vi "Dust_Type_Menu.vi"(8 "error in (no error)":errorcluster, 10 "Small?":bool, 11 "Enable":bool=TRUE) -> (0 "error out":errorcluster, 1 "Action Taken":T6(ring), 2 "Dust Properties":T3, 3 "Dust Info":T4 {"Batch" step=1; "Type" step=1; "Dust Source Builder:" items=["Keith Drake", "Nick Beaty", "Anthony Shu", "David James", "John Fontanese"]})   [LabVIEW 2015]
doc: "Displays a standard dialog box that prompts users to enter information, such as a user name and password.\n--------------------\n\nThis Express VI is configured as follows:\n\nMessage to Display to the User:Please Enter Experiment Settings Information For Database Storage.\nThe inputs are: \nNumber: Please Enter Group ID\nText Entry Box: Please Enter Tags:\nText Entry Box: Please Enter Experiment Description:"
uses:
  Controls/Dust_Properties.ctl
  Controls/source_builders.ctl
  Controls/dust_type_indicator.ctl
  Controls/Dust_list.ctl
  <vilib>/Utility/miscctls.llb/LVPointTypeDef.ctl
  <vilib>/Utility/error.llb/DialogType.ctl
  <userlib>/_OpenG.lib/array/array.llb/Remove Duplicates from 1D Array (String)__ogtk.vi
  <userlib>/_OpenG.lib/array/array.llb/Search 1D Array (String)__ogtk.vi
  <userlib>/_OpenG.lib/array/array.llb/Index 1D Array Elements (String)__ogtk.vi
  <vilib>/addons/database/_DB Variant To Data/Database Variant To Data.xnode
panel:
  out "Update Query":string
  out "Maxes Array":T1(array[cluster])
  out "All Dust Types":T2[](array[typedef])
  in  "Transfer":bool caption="OK2"
  in  "Controls":T4={"Dust info id"=0, "Integer Timestamp"=0, "Dust:"="", "Dust Source Builder:"=0, "Notes:"="", "Date of last dust source change:"=timestamp(0 s since 1904-01-01), "Initial Dust Mass:"=0.0, "Final Dust Mass:"=0.0, "Type"=0, "Batch"=1, "dust type id"=0, "Transferred?"=FALSE} {"Batch" min=1 max=2 step=1; "Type" min=1 max=1 step=1; "Dust Source Builder:" items=["Keith Drake", "Nick Beaty", "Anthony Shu", "David James", "John Fontanese"]}
  in  "Create New":bool caption="OK2"
  in  "Cancel":bool
  in  "Update":bool caption="OK1"
  # "Please Enter Dust Information For Storage in the CCLDAS Database."
  # "Dust Information"
  # "Dust Information"
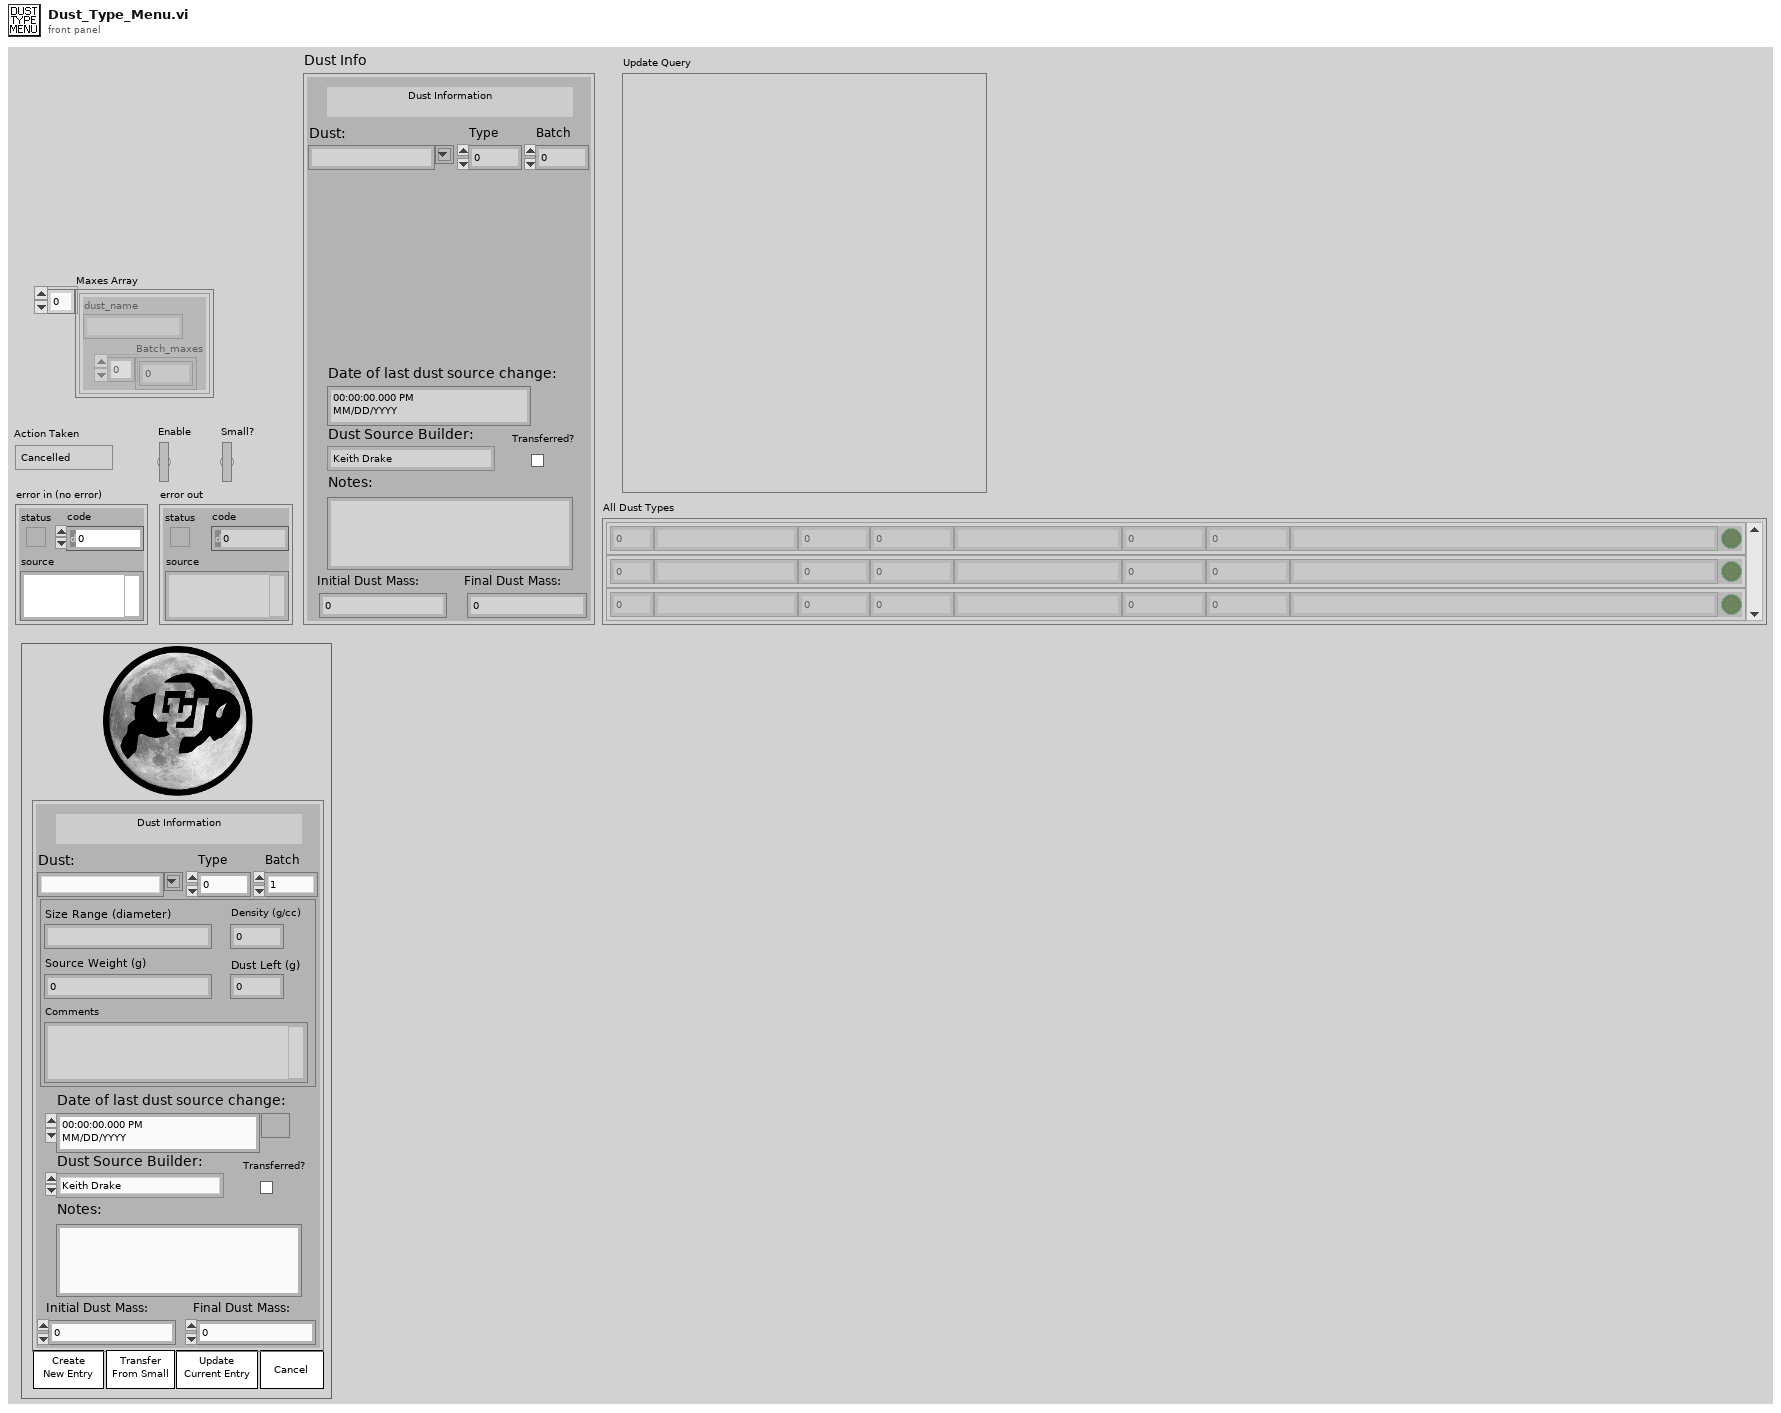
[diagram p1: front panel]
types:
  T1 = cluster{"dust_name":string, "Batch_maxes":i32[]}[]
  T2 = typedef "Dust_list.ctl" = cluster{"id_dust_type":i32, "dust_name":string, "dust_type":i32, "batch_no":i32, "dust_density":dbl, "source_weight":dbl, "size":string, "bottle_weight":dbl, "dust_mass":dbl, "comments":string, "Shoots?":bool}
  T3 = typedef "dust_type_indicator.ctl" = cluster{"id_dust_type":i32, "Size Range (diameter)":string, "Density (g/cc)":dbl, "Source Weight (g)":dbl, "Dust Left (g)":dbl, "Comments":string}
  T4 = typedef "Dust_Properties.ctl" = cluster{"Dust info id":u16, "Integer Timestamp":i64, "Dust:":string, "Dust Source Builder:":T5, "Notes:":string, "Date of last dust source change:":timestamp, "Initial Dust Mass:":dbl, "Final Dust Mass:":dbl, "Type":u16, "Batch":u16, "dust type id":u16, "Transferred?":bool}
  T5 = typedef "source_builders.ctl" = u16
  T6 = enum16{"Cancelled", "New", "Updated", "Transferred"}
  T7 = typedef "LVPointTypeDef.ctl" = cluster{"Horizontal":i16, "Vertical":i16}
  T8 = enum8{"Enabled", "Disabled", "Disabled and Grayed Out"}
  T9 = typedef "DialogType.ctl" = u16
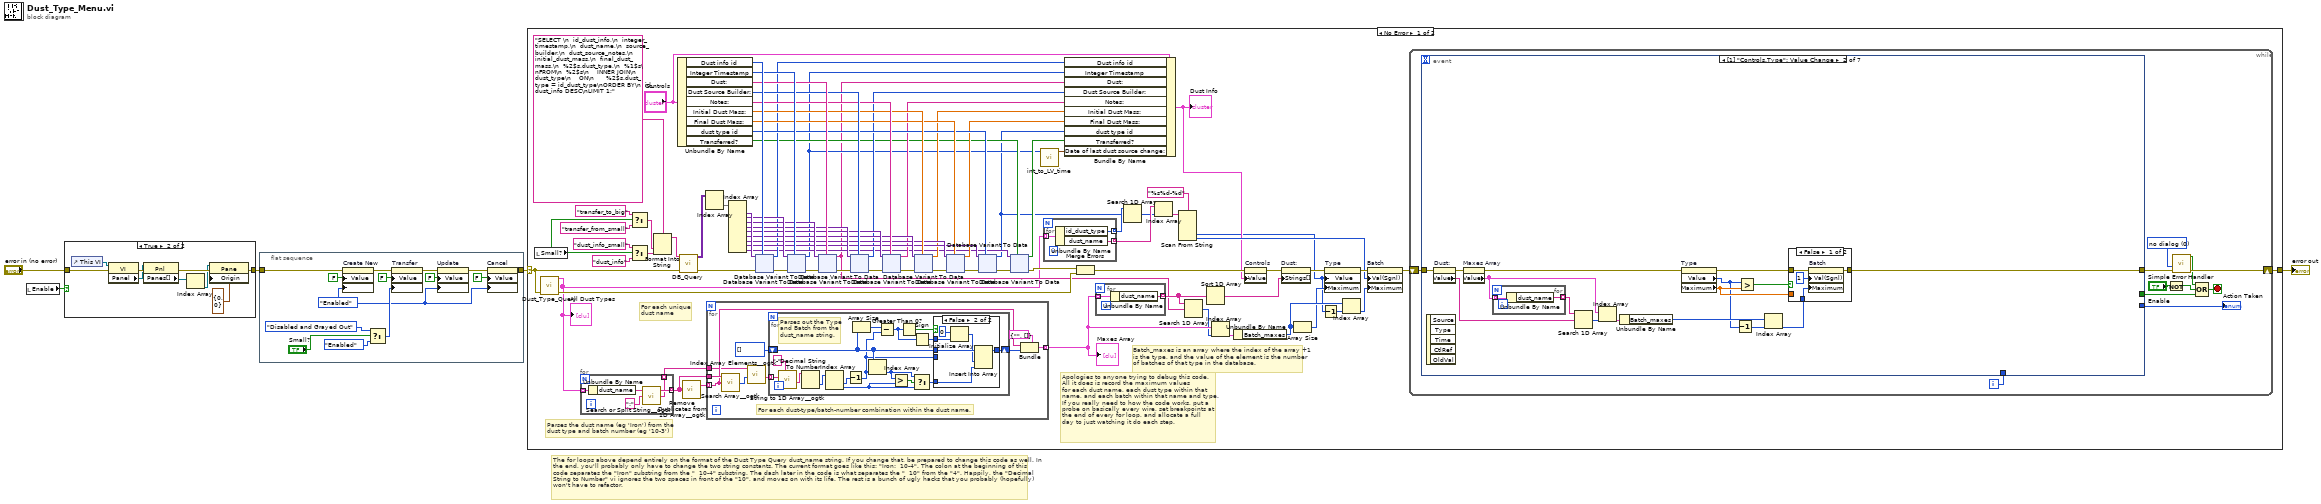
[diagram p0: block diagram]
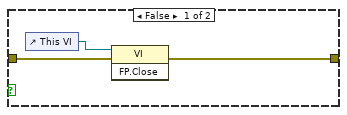
[diagram p2: hidden frame]
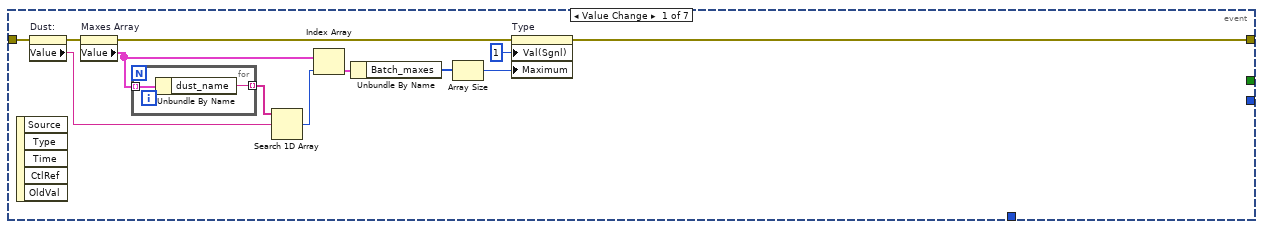
[diagram p3: hidden frame]
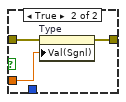
[diagram p4: hidden frame]
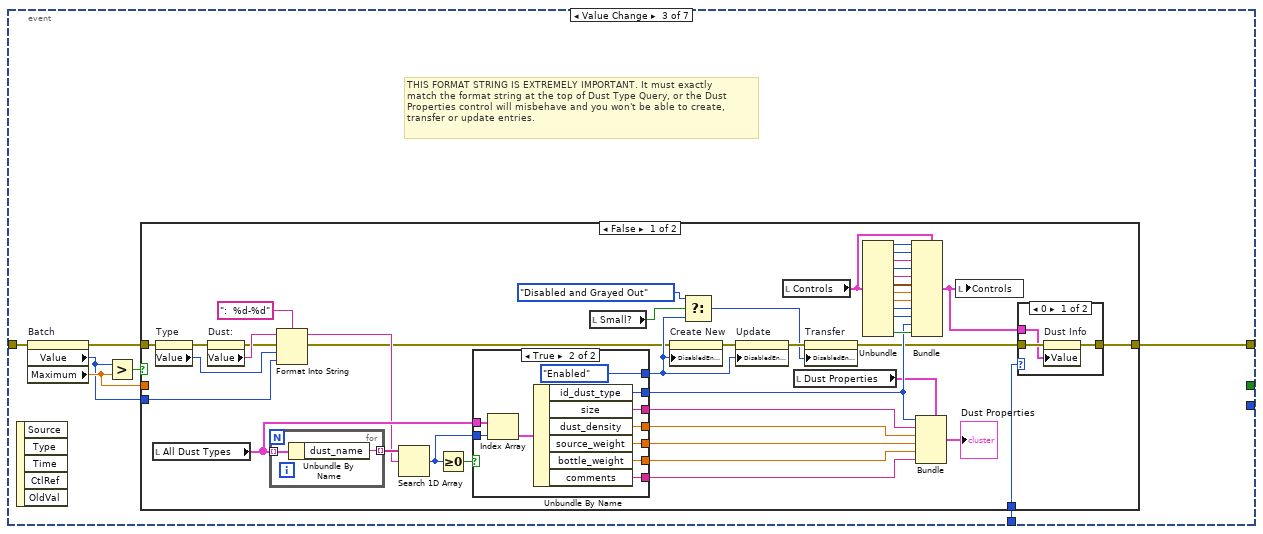
[diagram p5: hidden frame]
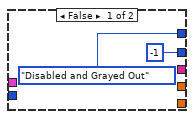
[diagram p7: hidden frame]
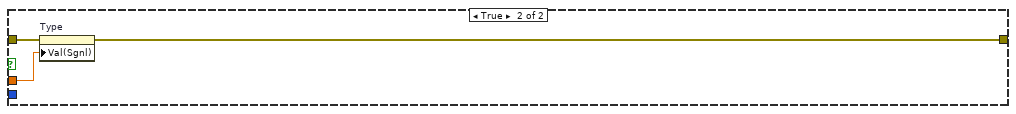
[diagram p8: hidden frame]
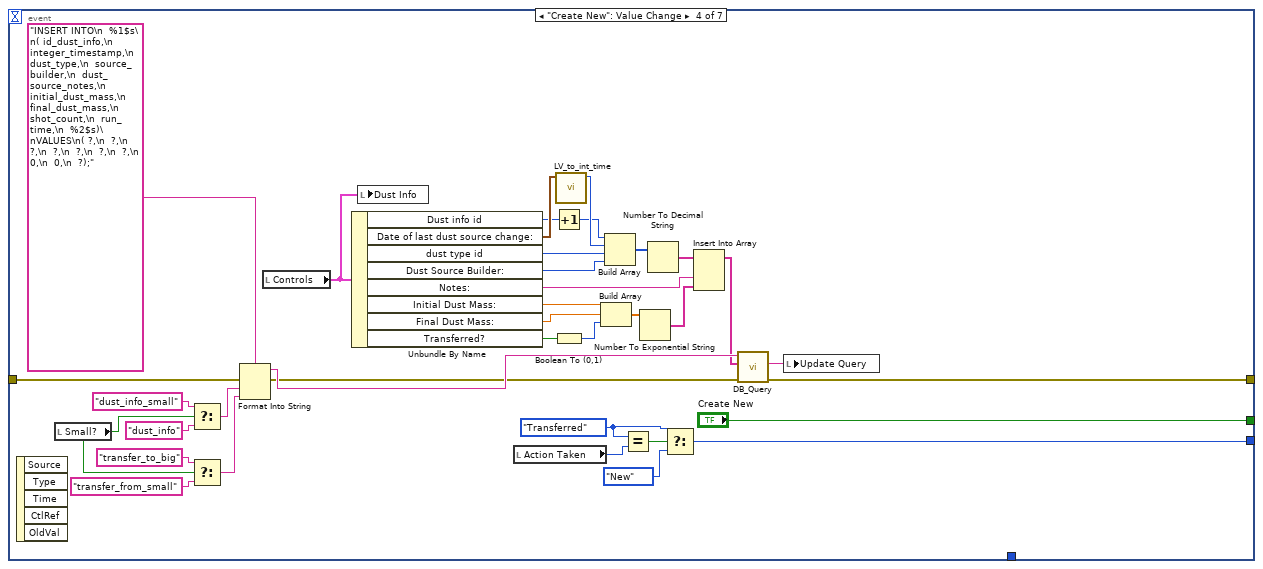
[diagram p9: hidden frame]
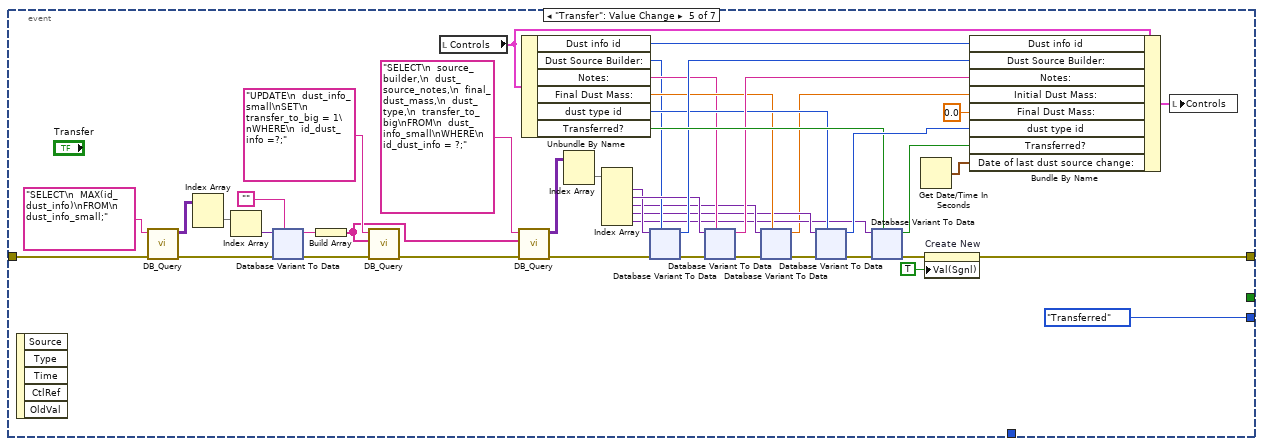
[diagram p10: hidden frame]
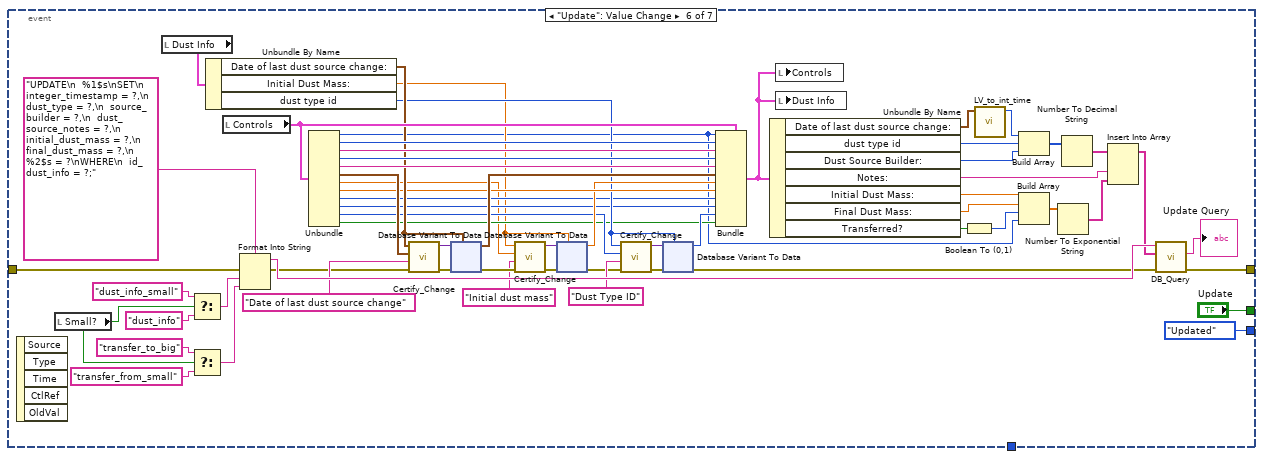
[diagram p11: hidden frame]
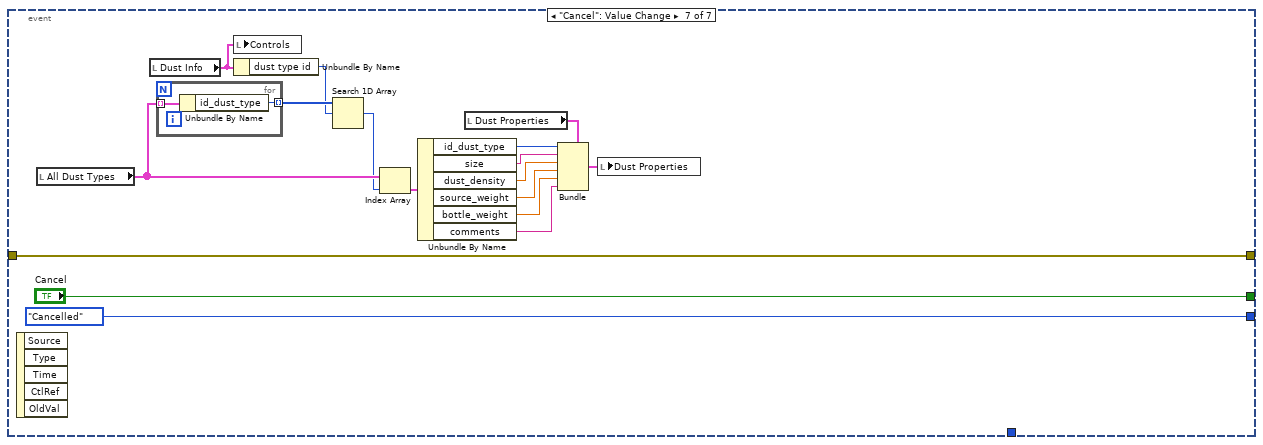
[diagram p12: hidden frame]
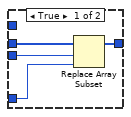
[diagram p13: hidden frame]
diagram:
  # "The for loops above depend entirely on the format of the Dust Type Query dust_name string. If you change that, be prepared to change this code as well. In\nthe end, you'll probably only have to change the two string constants. The current format goes like this: \"Iron:  10-4\". The colon at the beginning of this\ncode separates the \"Iron\" substring from the \"  10-4\" substring. The dash later in the code is what separates the \"  10\" from the \"4\". Happily, the \"Decimal\nString to Number\" vi ignores the two spaces in front of the \"10\", and moves on with its life. The rest is a bunch of ugly hacks that you probably (hopefully)\nwon't have to refactor."
  n1 = local read "Enable"() -> (w1:bool)
  n2 = case shown="True" w1 {
    tunnel: "error in (no error)" -> [w7 w10]
    tunnel: [w6 w9] -> w2
    frame False {
      n3 = control-ref of="This VI"() -> (w8:refnum<vi>)
      n4 = invoke class="VI" method="FP.Close"(reference=w8, error in=w7) -> (error out=w6:errorcluster)  [unwired: 1 in, 2 out]
    }
    frame True {
      n5 = control-ref of="This VI"() -> (w17:refnum<vi>)
      n6 = property class="VI"(reference=w17, error in=w10) -> (error out=w16:errorcluster, "Panel"=w15:refnum<vi>)  [unwired: 1 out]
      n7 = property class="Pnl"(reference=w15, error in=w16) -> (error out=w14:errorcluster, "Panes[]"=w13:refnum<vi>[])  [unwired: 1 out]
      n8 = Index Array(array=w13) -> (element=w12:refnum<vi>)  [unwired: 1 in]
      n9 = property class="Pane"(reference=w12, error in=w14, "Origin"=T7 {"Horizontal"=0, "Vertical"=0}) -> (error out=w9:errorcluster)  [unwired: 1 out]
    }
  }
  n10 = flat-sequence {
    tunnel: [w25] -> w3
    tunnel: w2 -> [w20]
    frame #0 {
      w18 = T8."Enabled" ("Disabled")
      n11 = property on="Create New" class="Bool (strict)"(error in=w20, "Value"=FALSE ("Create New"), "DisabledEnum"=w18) -> (error out=w26:errorcluster)  [unwired: 1 in, 1 out]
      n12 = Select(t=T8."Disabled and Grayed Out" ("Disabled"), s="Small?", f=T8."Enabled" ("Disabled")) -> (s? t:f=w19:T8)
      n13 = property on="Transfer" class="Bool (strict)"(error in=w26, "Value"=FALSE ("Transfer"), "DisabledEnum"=w19) -> (error out=w28:errorcluster)  [unwired: 1 in, 1 out]
      n14 = property on="Update" class="Bool (strict)"(error in=w28, "Value"=FALSE ("Update"), "DisabledEnum"=w18) -> (error out=w27:errorcluster)  [unwired: 1 in, 1 out]
      n15 = property on="Cancel" class="Bool (strict)"(error in=w27, "Value"=FALSE ("Cancel"), "DisabledEnum"=w18) -> (error out=w25:errorcluster)  [unwired: 1 in, 1 out]
    }
  }
  n16 = case shown="No Error" w3 {
    selector: w3 -> [w64 w1027]
    tunnel: [w55 w1027] -> w5
    frame No Error {
      # "Batch_maxes is an array where the index of the array +1\nis the type, and the value of the element is the number\nof batches of that type in the database."
      # "For each unique\ndust name"
      # "Parses the dust name (eg 'Iron') from the\ndust type and batch number (eg '10-3')"
      # "Apologies to anyone trying to debug this code.\nAll it does is record the maximum values\nfor each dust name, each dust type within that\nname, and each batch within that name and type.\nIf you really need to how the code works, put a\nprobe on basically every wire, set breakpoints at\nthe end of every for loop, and allocate a full\nday to just watching it do each step."
      n17 = local read "Small?"() -> (w102:bool)
      n18 = call "Dust_Type_Query.vi"("error in (no error)"=w64) -> ("error out"=w63:errorcluster, "Dust Type Array"=w43:T2[])  [unwired: 9 in]
      "All Dust Types" <- w43
      n19 = for {
        tunnel: w43 -> [w738] mode=indexing
        tunnel: [w736] -> w60 mode=indexing
        tunnel: [w734] -> w61 mode=indexing
        n20 = Unbundle By Name(w738) -> ("dust_name"=w735:string)
        n21 = call <userlib>:"Search or Split String__ogtk.vi"("search string/char (-)"=":", "string"=w735) -> ("substring after match"=w734:string, "substring before match"=w736:string)  [unwired: 1 in, 1 out]
      }
      n22 = Select(t="transfer_to_big", s=w102, f="transfer_from_small") -> (s? t:f=w103:string)
      n23 = Select(t="dust_info_small", s=w102, f="dust_info") -> (s? t:f=w107:string)
      n24 = Format Into String(format string="SELECT \n  id_dust_info,\n  integer_timestamp,\n  dust_name,\n  source_builder,\n  dust_source_notes,\n  initial_dust_mass,\n  final_dust_mass,\n  %2$s.dust_type,\n  %1$s\nFROM\n  %2$s\n    INNER JOIN\n  dust_type\n    ON\n      %2$s.dust_type = id_dust_type\nORDER BY\n  id_dust_info DESC\nLIMIT 1;" ("SQL query"), w103, w107) -> (resulting string=w106:string)  [unwired: 2 in, 1 out]
      n25 = Unbundle By Name("Controls") -> ("Dust info id"=w97:u16, "Integer Timestamp"=w94:i64, "Dust:"=w91:string, "Dust Source Builder:"=w89:T5, "Notes:"=w86:string, "Initial Dust Mass:"=w83:dbl, "Final Dust Mass:"=w79:dbl, "dust type id"=w76:u16, "Transferred?"=w68:bool)
      n26 = call "DB_Query.vi"("error in (no error)"=w64, "Parameterized Query"=w106) -> ("error out"=w101:errorcluster, "Results"=w100:variant[][])  [unwired: 7 in, 1 out]
      n27 = call-poly <userlib>:"Remove Duplicates from 1D Array__ogtk.vi"("Input Array"=w60) -> ("Output Array"=w62:string[])  [unwired: 1 out]
      n28 = Index Array(array=w100) -> (element=w99:variant[])  [unwired: 2 in]
      n29 = for {
        tunnel: w62 -> [w705] mode=indexing
        tunnel: w61 -> [w703]
        tunnel: w60 -> [w707]
        tunnel: [w699] -> w50 mode=indexing
        # "For each dust-type/batch-number combination within the dust name."
        n30 = call-poly <userlib>:"Search Array__ogtk.vi"("Array"=w707, "Element Data"=w705) -> ("Indices of Elements"=w704:i32[])  [unwired: 7 in]
        n31 = call-poly <userlib>:"Index Array Elements__ogtk.vi"("indices"=w704, "array"=w703) -> ("elements"=w702:string[])  [unwired: 9 in]
        n32 = for {
          tunnel: w702 -> [w720] mode=indexing
          shift-right: [w718] -> w700
          shift-left: i32[] [] ("array") -> [w713]
          # "Parses out the Type\nand Batch from the\ndust_name string."
          n33 = call <userlib>:"String to 1D Array__ogtk.vi"("delimiter (Tab)"="-", "string"=w720) -> ("Array of Strings"=w722:string[])  [unwired: 9 in]
          n34 = Decimal String To Number(string=w722) -> (number=w721:i32[])  [unwired: 2 in, 1 out]
          n35 = Index Array(array=w721) -> (element #1=w719:i32, element #2=w715:i32)  [unwired: 2 in]
          n36 = Decrement(x=w719) -> (x-1=w711:i32)
          n37 = Array Size(array=w713) -> (size(s)=w712:i32)
          n38 = Index Array(array=w713, index=w711) -> (element=w716:i32)
          n39 = Subtract(x=w712, y=w711) -> (x-y=w709:i32)
          n40 = Greater?(x=w716, y=w715) -> (0:w717:bool)
          n41 = Greater Than 0?(x=w709) -> (x > 0?=w710:bool)
          n42 = Select(t=w716, s=w717, f=w715) -> (s? t:f=w714:i32)
          n43 = Sign(1:w709) -> (0:w708:i32)
          n44 = case shown="False" w710 {
            tunnel: [w727 w733] -> w718
            tunnel: w713 -> [w726 w732]
            tunnel: w711 -> [w725 _]
            tunnel: w714 -> [w724 w731]
            tunnel: w708 -> [_ w730]
            frame True {
              n45 = Replace Array Subset(array=w726, new element=w724, index=w725) -> (w727:i32[])
            }
            frame False {
              n46 = Initialize Array(0 ("element"), w730) -> (w728:i32[])
              n47 = Insert Into Array(array=w732, new element #1=w728, new element #2=w731) -> (w733:i32[])  [unwired: 1 in]
            }
          }
        }
        n48 = Bundle(cluster=cluster{"dust_name":string, "Batch_maxes":i32[]} {"dust_name"="", "Batch_maxes"=[]}, "dust_name"=w705, "Batch_maxes"=w700) -> (w699:cluster{"dust_name":string, "Batch_maxes":i32[]})
      }
      "Maxes Array" <- w50
      n49 = Index Array(array=w99) -> (element #1=w98:variant, element #2=w95:variant, element #3=w92:variant, element #4=w88:variant, element #5=w85:variant, element #6=w82:variant, element #7=w80:variant, element #8=w77:variant, element #9=w66:variant)  [unwired: 9 in]
      n50 = xnode "Database Variant To Data"("database variant"=w98, "error in (no error)"=w101, "type"=w97) -> ("data"=w74:u16, "error out"=w96:errorcluster)
      n51 = xnode "Database Variant To Data"("database variant"=w95, "error in (no error)"=w96, "type"=w94) -> ("data"=w53:i64, "error out"=w93:errorcluster)
      n52 = xnode "Database Variant To Data"("database variant"=w92, "error in (no error)"=w93, "type"=w91) -> ("data"=w45:string, "error out"=w90:errorcluster)
      n53 = xnode "Database Variant To Data"("database variant"=w88, "error in (no error)"=w90, "type"=w89) -> ("data"=w73:T5, "error out"=w87:errorcluster)
      n54 = xnode "Database Variant To Data"("database variant"=w85, "error in (no error)"=w87, "type"=w86) -> ("data"=w72:string, "error out"=w84:errorcluster)
      n55 = xnode "Database Variant To Data"("database variant"=w82, "error in (no error)"=w84, "type"=w83) -> ("data"=w71:dbl, "error out"=w81:errorcluster)
      n56 = xnode "Database Variant To Data"("database variant"=w80, "error in (no error)"=w81, "type"=w79) -> ("data"=w70:dbl, "error out"=w78:errorcluster)
      n57 = xnode "Database Variant To Data"("database variant"=w77, "error in (no error)"=w78, "type"=w76) -> ("data"=w41:u16, "error out"=w69:errorcluster)
      n58 = xnode "Database Variant To Data"("database variant"=w66, "error in (no error)"=w69, "type"=w68) -> ("data"=w67:bool, "error out"=w65:errorcluster)
      n59 = call "int_to_LV_time.vi"("Integer Timestamp"=w53) -> ("time stamp"=w54:timestamp)  [unwired: 8 in, 1 out]
      n60 = for {
        tunnel: w43 -> [w113] mode=indexing
        tunnel: [w112] -> w42 mode=indexing
        tunnel: [w111] -> w40 mode=indexing
        n61 = Unbundle By Name(w113) -> ("id_dust_type"=w112:i32, "dust_name"=w111:string)
      }
      n62 = Bundle By Name(cluster="Controls", "Dust info id"=w74, "Integer Timestamp"=w53, "Dust:"=w45, "Dust Source Builder:"=w73, "Notes:"=w72, "Initial Dust Mass:"=w71, "Final Dust Mass:"=w70, "dust type id"=w41, "Transferred?"=w67, "Date of last dust source change:"=w54) -> (w33:T4)
      "Dust Info" <- w33
      n63 = Merge Errors(w65, w63) -> (w34:errorcluster)
      n64 = for {
        tunnel: w50 -> [w698] mode=indexing
        tunnel: [w697] -> w49 mode=indexing
        n65 = Unbundle By Name(w698) -> ("dust_name"=w697:string)
      }
      n66 = Search 1D Array(1D array=w42, element=w41) -> (index of element=w39:i32)  [unwired: 1 in]
      n67 = Index Array(array=w40, index=w39) -> (element=w38:string)
      n68 = Scan From String(format string="%s%d-%d", input string=w38) -> (output 2=w32:i32, output 3=w36:i32)  [unwired: 6 in, 3 out]
      n69 = Search 1D Array(1D array=w49, element=w45) -> (index of element=w48:i32)  [unwired: 1 in]
      n70 = Sort 1D Array(array=w49) -> (sorted array=w52:string[])
      n71 = Index Array(array=w50, index=w48) -> (element=w59:cluster{"dust_name":string, "Batch_maxes":i32[]})
      n72 = Unbundle By Name(w59) -> ("Batch_maxes"=w58:i32[])
      n73 = property on="Controls" class="Clust (strict)"(error in=w34, "Value"=w33) -> (error out=w35:errorcluster)  [unwired: 1 in, 1 out]
      n74 = property on="Dust:" class="CmbBox"(error in=w35, "Strings[]"=w52) -> (error out=w56:errorcluster)  [unwired: 1 in, 1 out]
      n75 = Array Size(array=w58) -> (size(s)=w46:i32)
      n76 = Decrement(x=w32) -> (x-1=w47:i32)
      n77 = property on="Type" class="DigNum (strict)"(error in=w56, "Value"=w32, "Maximum"=w46) -> (error out=w57:errorcluster)  [unwired: 1 in, 1 out]
      n78 = Index Array(array=w58, index=w47) -> (element=w51:i32)
      n79 = property on="Batch" class="DigNum (strict)"(error in=w57, "Val(Sgnl)"=w36, "Maximum"=w51) -> (error out=w44:errorcluster)  [unwired: 1 in, 1 out]
      n80 = while {
        shift-right: [w120] -> w55
        shift-left: w44 -> [w124]
        i -> [w114]
        stop <- w118 stop-if-true
        w119 = T9 0 items=["no dialog", "OK message", "continue or stop message", "OK message + warnings", "continue/stop + warnings"] ("type of dialog (OK msg:1)")
        n81 = event shown="[1] \"Controls.Type\": Value Change" {
          selector: _ -> [_ _ _ _ _ _ _]
          dyn-events: _ -> [_ _ _ _ _ _ _]
          timeout: _ -> [_ _ _ _ _ _ _]
          tunnel: w124 -> [w136 w148 w167 w245 w281 w558 w693]
          tunnel: [w125 w145 w166 w247 w282 w544 w693] -> w123
          tunnel: [_ _ _ "Create New" _ "Update" "Cancel"] -> w122
          tunnel: [_ _ _ w235 T6."Transferred" ("Action Taken") T6."Updated" ("Action Taken") T6."Cancelled" ("Action Taken")] -> w121
          tunnel: w114 -> [_ _ w164 _ _ _ _]
          event Value Change {
            n82 = event-data() -> ()  [unwired: 1 in, 5 out]
            n83 = property on="Dust:" class="CmbBox"(error in=w136) -> (error out=w135:errorcluster, "Value"=w126:string)  [unwired: 1 in, 1 out]
            n84 = property on="Maxes Array" class="Arr (strict)"(error in=w135) -> (error out=w134:errorcluster, "Value"=w131:T1)  [unwired: 1 in, 1 out]
            n85 = for {
              tunnel: w131 -> [w138] mode=indexing
              tunnel: [w137] -> w133 mode=indexing
              n86 = Unbundle By Name(w138) -> ("dust_name"=w137:string)
            }
            n87 = Search 1D Array(1D array=w133, element=w126) -> (index of element=w127:i32)  [unwired: 1 in]
            n88 = Index Array(array=w131, index=w127) -> (element=w130:cluster{"dust_name":string, "Batch_maxes":i32[]})
            n89 = Unbundle By Name(w130) -> ("Batch_maxes"=w129:i32[])
            n90 = Array Size(array=w129) -> (size(s)=w128:i32)
            n91 = property on="Type" class="DigNum (strict)"(error in=w134, "Val(Sgnl)"=u16 1 ("Value"), "Maximum"=w128) -> (error out=w125:errorcluster)  [unwired: 1 in, 1 out]
          }
          event Value Change {
            n92 = event-data() -> ()  [unwired: 1 in, 5 out]
            n93 = property on="Dust:" class="CmbBox"(error in=w148) -> (error out=w154:errorcluster, "Value"=w152:string)  [unwired: 1 in, 1 out]
            n94 = property on="Maxes Array" class="Arr (strict)"(error in=w154) -> (error out=w142:errorcluster, "Value"=w150:T1)  [unwired: 1 in, 1 out]
            n95 = for {
              tunnel: w150 -> [w163] mode=indexing
              tunnel: [w162] -> w153 mode=indexing
              n96 = Unbundle By Name(w163) -> ("dust_name"=w162:string)
            }
            n97 = Search 1D Array(1D array=w153, element=w152) -> (index of element=w151:i32)  [unwired: 1 in]
            n98 = Index Array(array=w150, index=w151) -> (element=w149:cluster{"dust_name":string, "Batch_maxes":i32[]})
            n99 = Unbundle By Name(w149) -> ("Batch_maxes"=w141:i32[])
            n100 = property on="Type" class="DigNum (strict)"(error in=w142) -> (error out=w147:errorcluster, "Value"=w140:u16, "Maximum"=w146:dbl)  [unwired: 1 in, 1 out]
            n101 = Decrement(x=w140) -> (x-1=w139:u16)
            n102 = Greater?(x=w140, y=w146) -> (0:w144:bool)
            n103 = Index Array(array=w141, index=w139) -> (element=w143:i32)
            n104 = case shown="False" w144 {
              tunnel: w147 -> [w157 w161]
              tunnel: w146 -> [_ w160]
              tunnel: [w156 w159] -> w145
              tunnel: w143 -> [w155 _]
              frame False {
                n105 = property on="Batch" class="DigNum (strict)"(error in=w157, "Val(Sgnl)"=u16 1 ("Value (Signaling)"), "Maximum"=w155) -> (error out=w156:errorcluster)  [unwired: 1 in, 1 out]
              }
              frame True {
                n106 = property on="Type" class="DigNum (strict)"(error in=w161, "Val(Sgnl)"=w160) -> (error out=w159:errorcluster)  [unwired: 1 in, 1 out]
              }
            }
          }
          event Value Change {
            # "THIS FORMAT STRING IS EXTREMELY IMPORTANT. It must exactly\nmatch the format string at the top of Dust Type Query, or the Dust\nProperties control will misbehave and you won't be able to create,\ntransfer or update entries."
            n107 = event-data() -> ()  [unwired: 1 in, 5 out]
            n108 = property on="Batch" class="DigNum (strict)"(error in=w167) -> (error out=w170:errorcluster, "Value"=w165:u16, "Maximum"=w169:dbl)  [unwired: 1 in, 1 out]
            n109 = Greater?(x=w165, y=w169) -> (0:w168:bool)
            n110 = case shown="False" w168 {
              tunnel: w170 -> [w208 w234]
              tunnel: w169 -> [_ w233]
              tunnel: [w174 w232] -> w166
              tunnel: w165 -> [w207 _]
              tunnel: w164 -> [w171 _]
              frame False {
                n111 = local read "All Dust Types"() -> (w213:T2[])
                n112 = property on="Type" class="DigNum (strict)"(error in=w208) -> (error out=w209:errorcluster, "Value"=w205:u16)  [unwired: 1 in, 1 out]
                n113 = property on="Dust:" class="CmbBox"(error in=w209) -> (error out=w177:errorcluster, "Value"=w206:string)  [unwired: 1 in, 1 out]
                n114 = for {
                  tunnel: w213 -> [w231] mode=indexing
                  tunnel: [w230] -> w212 mode=indexing
                  n115 = Unbundle By Name(w231) -> ("dust_name"=w230:string)
                }
                n116 = Format Into String(format string=":  %d-%d", initial string=w206, error in=w177, w205, w207) -> (resulting string=w210:string, error out=w176:errorcluster)
                n117 = Search 1D Array(1D array=w212, element=w210) -> (index of element=w185:i32)  [unwired: 1 in]
                n118 = Greater Or Equal To 0?(x=w185) -> (x >= 0?=w186:bool)
                n119 = case shown="True" w186 {
                  tunnel: w213 -> [_ w228]
                  tunnel: w185 -> [_ w227]
                  tunnel: [_ w226] -> w204
                  tunnel: [_ w225] -> w203
                  tunnel: [_ w224] -> w202
                  tunnel: [_ w223] -> w201
                  tunnel: [_ w222] -> w200
                  tunnel: [-1 ("id_dust_type") w221] -> w187
                  tunnel: [T8."Disabled and Grayed Out" ("Disabled") T8."Enabled" ("Disabled")] -> w179
                  frame False {
                  }
                  frame True {
                    n120 = Index Array(array=w228, index=w227) -> (element=w229:T2)
                    n121 = Unbundle By Name(w229) -> ("id_dust_type"=w221:i32, "size"=w226:string, "dust_density"=w225:dbl, "source_weight"=w224:dbl, "bottle_weight"=w223:dbl, "comments"=w222:string)
                  }
                }
                n122 = local read "Small?"() -> (w180:bool)
                n123 = property on="Create New" class="Bool (strict)"(error in=w176, "DisabledEnum"=w179) -> (error out=w182:errorcluster)  [unwired: 1 in, 1 out]
                n124 = Select(t=T8."Disabled and Grayed Out" ("Disabled"), s=w180, f=w179) -> (s? t:f=w178:T8)
                n125 = property on="Update" class="Bool (strict)"(error in=w182, "DisabledEnum"=w179) -> (error out=w183:errorcluster)  [unwired: 1 in, 1 out]
                n126 = local read "Controls"() -> (w199:T4)
                n127 = local read "Dust Properties"() -> (w184:T3)
                n128 = property on="Transfer" class="Bool (strict)"(error in=w183, "DisabledEnum"=w178) -> (error out=w172:errorcluster)  [unwired: 1 in, 1 out]
                n129 = Unbundle(w199) -> ("Dust info id"=w198:u16, "Integer Timestamp"=w197:i64, "Dust:"=w196:string, "Dust Source Builder:"=w195:T5, "Notes:"=w194:string, "Date of last dust source change:"=w193:timestamp, "Initial Dust Mass:"=w192:dbl, "Final Dust Mass:"=w191:dbl, "Type"=w190:u16, "Batch"=w189:u16, "Transferred?"=w188:bool)  [unwired: 1 out]
                n130 = Bundle(cluster=w199, "Dust info id"=w198, "Integer Timestamp"=w197, "Dust:"=w196, "Dust Source Builder:"=w195, "Notes:"=w194, "Date of last dust source change:"=w193, "Initial Dust Mass:"=w192, "Final Dust Mass:"=w191, "Type"=w190, "Batch"=w189, "dust type id"=w187, "Transferred?"=w188) -> (w173:T4)
                n131 = Bundle(cluster=w184, "id_dust_type"=w187, "Size Range (diameter)"=w204, "Density (g/cc)"=w203, "Source Weight (g)"=w202, "Dust Left (g)"=w201, "Comments"=w200) -> (→"Dust Properties":T3)
                n132 = local write "Controls"(w173) -> ()
                n133 = case shown="0" w171 {
                  tunnel: w172 -> [w216 w217]
                  tunnel: [w215 w217] -> w174
                  tunnel: w173 -> [w214 _]
                  frame 0 {
                    n134 = property on="Dust Info" class="Clust (strict)"(error in=w216, "Value"=w214) -> (error out=w215:errorcluster)  [unwired: 1 in, 1 out]
                  }
                  frame Default {
                  }
                }
              }
              frame True {
                n135 = property on="Type" class="DigNum (strict)"(error in=w234, "Val(Sgnl)"=w233) -> (error out=w232:errorcluster)  [unwired: 1 in, 1 out]
              }
            }
          }
          event "Create New": Value Change {
            w237 = T6."Transferred" ("Action Taken")
            n136 = event-data() -> ()  [unwired: 1 in, 5 out]
            n137 = local read "Small?"() -> (w267:bool)
            n138 = Select(t="dust_info_small", s=w267, f="dust_info") -> (s? t:f=w264:string)
            n139 = Select(t="transfer_to_big", s=w267, f="transfer_from_small") -> (s? t:f=w263:string)
            n140 = Format Into String(format string="INSERT INTO\n  %1$s\n( id_dust_info,\n  integer_timestamp,\n  dust_type,\n  source_builder,\n  dust_source_notes,\n  initial_dust_mass,\n  final_dust_mass,\n  shot_count,\n  run_time,\n  %2$s)\nVALUES\n( ?,\n  ?,\n  ?,\n  ?,\n  ?,\n  ?,\n  ?,\n  0,\n  0,\n  ?);", error in=w245, w264, w263) -> (resulting string=w268:string, error out=w243:errorcluster)  [unwired: 1 in]
            n141 = local read "Controls"() -> (w244:T4)
            n142 = Unbundle By Name(w244) -> ("Dust info id"=w242:u16, "Date of last dust source change:"=w262:timestamp, "dust type id"=w259:u16, "Dust Source Builder:"=w248:T5, "Notes:"=w249:string, "Initial Dust Mass:"=w257:dbl, "Final Dust Mass:"=w256:dbl, "Transferred?"=w261:bool)
            n143 = local write "Dust Info"(w244) -> ()
            n144 = local read "Action Taken"() -> (w238:T6)
            n145 = Increment(x=w242) -> (x+1=w241:u16)
            n146 = Boolean To (0,1)(Boolean=w261) -> (0, 1=w255:i16)
            n147 = call "LV_to_int_time.vi"("Time Stamp"=w262) -> ("Integer Time"=w260:i64)  [unwired: 8 in, 1 out]
            n148 = Build Array(w257, w256, w255) -> (w254:dbl[])
            n149 = Build Array(w241, w260, w259, w248) -> (w258:i64[])
            n150 = Equal?(x=w237, y=w238) -> (x = y?=w239:bool)
            n151 = Number To Exponential String(number=w254) -> (E-format string=w252:string[])  [unwired: 3 in]
            n152 = Number To Decimal String(number=w258) -> (decimal integer string=w253:string[])  [unwired: 1 in]
            n153 = Select(t=w237, s=w239, f=T6."New" ("Action Taken")) -> (s? t:f=w235:T6)
            n154 = Insert Into Array(array=w253, new element #1=w249, new element #2=w252) -> (w251:string[])  [unwired: 1 in]
            n155 = call "DB_Query.vi"("error in (no error)"=w243, "Parameters"=w251, "Parameterized Query"=w268) -> ("error out"=w247:errorcluster, "Query in Standard Format"=w246:string)  [unwired: 6 in, 1 out]
            n156 = local write "Update Query"(w246) -> ()
          }
          event "Transfer": Value Change {
            n157 = event-data() -> ()  [unwired: 1 in, 5 out]
            n158 = call "DB_Query.vi"("error in (no error)"=w281, "Parameterized Query"="SELECT\n  MAX(id_dust_info)\nFROM\n  dust_info_small;") -> ("error out"=w275:errorcluster, "Results"=w279:variant[][])  [unwired: 7 in, 1 out]
            n159 = Index Array(array=w279) -> (element=w278:variant[])  [unwired: 2 in]
            n160 = Index Array(array=w278) -> (element=w277:variant)  [unwired: 1 in]
            n161 = xnode "Database Variant To Data"("database variant"=w277, "error in (no error)"=w275, "type"="") -> ("data"=w273:string, "error out"=w274:errorcluster)
            n162 = Build Array(w273) -> (w272:string[])
            n163 = call "DB_Query.vi"("error in (no error)"=w274, "Parameters"=w272, "Parameterized Query"="UPDATE\n  dust_info_small\nSET\n  transfer_to_big = 1\nWHERE\n  id_dust_info =?;") -> ("error out"=w310:errorcluster)  [unwired: 6 in, 2 out]
            n164 = local read "Controls"() -> (w294:T4)
            n165 = call "DB_Query.vi"("error in (no error)"=w310, "Parameters"=w272, "Parameterized Query"="SELECT\n  source_builder,\n  dust_source_notes,\n  final_dust_mass,\n  dust_type,\n  transfer_to_big\nFROM\n  dust_info_small\nWHERE\n  id_dust_info = ?;") -> ("error out"=w285:errorcluster, "Results"=w312:variant[][])  [unwired: 6 in, 1 out]
            n166 = Unbundle By Name(w294) -> ("Dust info id"=w271:u16, "Dust Source Builder:"=w296:T5, "Notes:"=w299:string, "Final Dust Mass:"=w301:dbl, "dust type id"=w303:u16, "Transferred?"=w307:bool)
            n167 = Index Array(array=w312) -> (element=w295:variant[])  [unwired: 2 in]
            n168 = Index Array(array=w295) -> (element #1=w297:variant, element #2=w300:variant, element #3=w290:variant, element #4=w289:variant, element #5=w288:variant)  [unwired: 5 in]
            n169 = xnode "Database Variant To Data"("database variant"=w297, "error in (no error)"=w285, "type"=w296) -> ("data"=w304:T5, "error out"=w298:errorcluster)
            n170 = xnode "Database Variant To Data"("database variant"=w300, "error in (no error)"=w298, "type"=w299) -> ("data"=w305:string, "error out"=w291:errorcluster)
            n171 = xnode "Database Variant To Data"("database variant"=w290, "error in (no error)"=w291, "type"=w301) -> ("data"=w287:dbl, "error out"=w302:errorcluster)
            n172 = xnode "Database Variant To Data"("database variant"=w289, "error in (no error)"=w302, "type"=w303) -> ("data"=w309:u16, "error out"=w306:errorcluster)
            n173 = xnode "Database Variant To Data"("database variant"=w288, "error in (no error)"=w306, "type"=w307) -> ("data"=w308:bool, "error out"=w284:errorcluster)
            n174 = Get Date/Time In Seconds() -> (seconds since 1Jan1904=w293:timestamp)
            n175 = property on="Create New" class="Bool (strict)"(error in=w284, "Val(Sgnl)"=TRUE ("Value (Signaling)")) -> (error out=w282:errorcluster)  [unwired: 1 in, 1 out]
            n176 = Bundle By Name(cluster=w294, "Dust info id"=w271, "Dust Source Builder:"=w304, "Notes:"=w305, "Initial Dust Mass:"=w287, "Final Dust Mass:"=0.0, "dust type id"=w309, "Transferred?"=w308, "Date of last dust source change:"=w293) -> (w292:T4)
            n177 = local write "Controls"(w292) -> ()
          }
          event "Update": Value Change {
            n178 = event-data() -> ()  [unwired: 1 in, 5 out]
            n179 = local read "Small?"() -> (w564:bool)
            n180 = local read "Dust Info"() -> (w540:T4)
            n181 = Select(t="dust_info_small", s=w564, f="dust_info") -> (s? t:f=w560:string)
            n182 = Select(t="transfer_to_big", s=w564, f="transfer_from_small") -> (s? t:f=w559:string)
            n183 = Unbundle By Name(w540) -> ("Date of last dust source change:"=w529:timestamp, "Initial Dust Mass:"=w510:dbl, "dust type id"=w518:u16)
            n184 = local read "Controls"() -> (w535:T4)
            n185 = Format Into String(format string="UPDATE\n  %1$s\nSET\n  integer_timestamp = ?,\n  dust_type = ?,\n  source_builder = ?,\n  dust_source_notes = ?,\n  initial_dust_mass = ?,\n  final_dust_mass = ?,\n  %2$s = ?\nWHERE\n  id_dust_info = ?;", error in=w558, w560, w559) -> (resulting string=w566:string, error out=w533:errorcluster)  [unwired: 1 in]
            n186 = Unbundle(w535) -> ("Dust info id"=w508:u16, "Integer Timestamp"=w539:i64, "Dust:"=w538:string, "Dust Source Builder:"=w537:T5, "Notes:"=w536:string, "Date of last dust source change:"=w532:timestamp, "Initial Dust Mass:"=w509:dbl, "Final Dust Mass:"=w524:dbl, "Type"=w516:u16, "Batch"=w515:u16, "dust type id"=w517:u16, "Transferred?"=w513:bool)
            n187 = call "Certify_Change.vi"("error in (no error)"=w533, "Variable Name"="Date of last dust source change", "New Value"=w532, "Default Value"=w529) -> ("error out"=w531:errorcluster, "Value Out"=w530:variant)  [unwired: 6 in]
            n188 = xnode "Database Variant To Data"("database variant"=w530, "error in (no error)"=w531, "type"=w529) -> ("data"=w528:timestamp, "error out"=w525:errorcluster)
            n189 = call "Certify_Change.vi"("error in (no error)"=w525, "Variable Name"="Initial dust mass", "New Value"=w509, "Default Value"=w510) -> ("error out"=w526:errorcluster, "Value Out"=w527:variant)  [unwired: 6 in]
            n190 = xnode "Database Variant To Data"("database variant"=w527, "error in (no error)"=w526, "type"=w510) -> ("data"=w522:dbl, "error out"=w512:errorcluster)
            n191 = call "Certify_Change.vi"("error in (no error)"=w512, "Variable Name"="Dust Type ID", "New Value"=w517, "Default Value"=w518) -> ("error out"=w520:errorcluster, "Value Out"=w519:variant)  [unwired: 6 in]
            n192 = xnode "Database Variant To Data"("database variant"=w519, "error in (no error)"=w520, "type"=w518) -> ("data"=w514:u16, "error out"=w511:errorcluster)
            n193 = Bundle(cluster=w535, "Dust info id"=w508, "Integer Timestamp"=w539, "Dust:"=w538, "Dust Source Builder:"=w537, "Notes:"=w536, "Date of last dust source change:"=w528, "Initial Dust Mass:"=w522, "Final Dust Mass:"=w524, "Type"=w516, "Batch"=w515, "dust type id"=w514, "Transferred?"=w513) -> (w507:T4)
            n194 = Unbundle By Name(w507) -> ("Date of last dust source change:"=w557:timestamp, "dust type id"=w554:u16, "Dust Source Builder:"=w541:T5, "Notes:"=w542:string, "Initial Dust Mass:"=w552:dbl, "Final Dust Mass:"=w551:dbl, "Transferred?"=w556:bool)
            n195 = local write "Controls"(w507) -> ()
            n196 = local write "Dust Info"(w507) -> ()
            n197 = Boolean To (0,1)(Boolean=w556) -> (0, 1=w550:i16)
            n198 = call "LV_to_int_time.vi"("Time Stamp"=w557) -> ("Integer Time"=w555:i64)  [unwired: 8 in, 1 out]
            n199 = Build Array(w555, w554, w541) -> (w553:i64[])
            n200 = Build Array(w552, w551, w550, w508) -> (w549:dbl[])
            n201 = Number To Exponential String(number=w549) -> (E-format string=w547:string[])  [unwired: 3 in]
            n202 = Number To Decimal String(number=w553) -> (decimal integer string=w548:string[])  [unwired: 1 in]
            n203 = Insert Into Array(array=w548, new element #1=w542, new element #2=w547) -> (w546:string[])  [unwired: 1 in]
            n204 = call "DB_Query.vi"("error in (no error)"=w511, "Parameters"=w546, "Parameterized Query"=w566) -> ("error out"=w544:errorcluster, "Query in Standard Format"=→"Update Query":string)  [unwired: 6 in, 1 out]
          }
          event "Cancel": Value Change {
            n205 = event-data() -> ()  [unwired: 1 in, 5 out]
            n206 = local read "All Dust Types"() -> (w682:T2[])
            n207 = local read "Dust Info"() -> (w678:T4)
            n208 = for {
              tunnel: w682 -> [w696] mode=indexing
              tunnel: [w695] -> w681 mode=indexing
              n209 = Unbundle By Name(w696) -> ("id_dust_type"=w695:i32)
            }
            n210 = local write "Controls"(w678) -> ()
            n211 = Unbundle By Name(w678) -> ("dust type id"=w680:u16)
            n212 = Search 1D Array(1D array=w681, element=w680) -> (index of element=w679:i32)  [unwired: 1 in]
            n213 = Index Array(array=w682, index=w679) -> (element=w692:T2)
            n214 = Unbundle By Name(w692) -> ("id_dust_type"=w683:i32, "size"=w684:string, "dust_density"=w685:dbl, "source_weight"=w686:dbl, "bottle_weight"=w687:dbl, "comments"=w688:string)
            n215 = local read "Dust Properties"() -> (w691:T3)
            n216 = Bundle(cluster=w691, "id_dust_type"=w683, "Size Range (diameter)"=w684, "Density (g/cc)"=w685, "Source Weight (g)"=w686, "Dust Left (g)"=w687, "Comments"=w688) -> (w690:T3)
            n217 = local write "Dust Properties"(w690) -> ()
          }
        }
        "Action Taken" <- w121
        n218 = Not(x="Enable") -> (.not. x?=w115:bool)
        n219 = call <vilib>:"Simple Error Handler.vi"("type of dialog (OK msg:1)"=w119, "error in (no error)"=w123) -> ("error?"=w117:bool, "error out"=w120:errorcluster)  [unwired: 3 in, 3 out]
        n220 = Compound Arithmetic op=OR(w117, w115, w122) -> (w118:bool)
      }
    }
    frame Error {
    }
  }
  "error out" <- w5
